vi "FTW-Test.vi"() -> ()   [LabVIEW 2015]
uses:
  src/time/FTW-Time-DisplayFormat-Timestamp.ctl
  src/json/core/FTW-JSON-Core-Type.ctl
  src/reflection/FTW-Reflection-Types.ctl
  src/error/FTW-ERR-ExceptionType.ctl
  src/time/FTW-Time-RelativeTimer.vi
  codegen/xnode/json/fetch/FTW-JSON-Core-GetFlattenedValue.vi
  src/error/FTW-ERR-ThrowInvalidReferenceError.vi
  src/json/core/FTW-JSON-Core-ElementType.vi
  codegen/xnode/FTW-Dataflow-Synchronizer.xnode
  codegen/xnode/FTW-JSON-Fetch.xnode
  codegen/xnode/FTW-Array-Shuffle.xnode
  src/json/FTW-JSON-Type.ctl
panel:
  out "Results":string
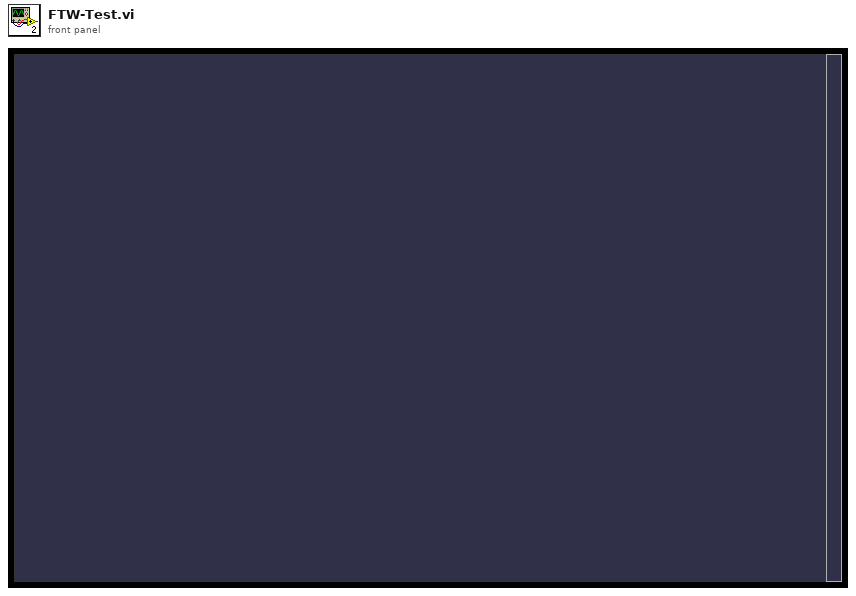
[diagram p1: front panel]
types:
  T1 = typedef "FTW-Time-DisplayFormat-Timestamp.ctl" = enum16{"YYYY-MM-DDT00:00:00.000Z (ISO-8601)", "YYYY-MM-DDT00-00-00Z (Simple ISO-8601)", "YYYY-MM-DD"}
  T2 = cluster{"Randomize Test Order":bool, "Tests Directory":path, "Test Configuration":cluster{"Default":cluster{"Enable":bool, "Iterations":i32}}, "Test Configuration":string, "Test Worker Pool Size":i32}
  T3 = typedef "FTW-Type-JSON.ctl" = refnum<data-value>
  T4 = enum32{"invalid app kind", "Development System", "Run Time System", "Student Edition", "Embedded LabVIEW", "Evaluation", "Custom"}
  T5 = enum32{"invalid CPU target", "Motorola 68K", "PowerPC", "Intel x86", "SPARC", "PA-RISC", "MIPS", "Alpha", "ARM", "AMD/Intel x64"}
  T6 = typedef "FTW-JSON-Core-Type.ctl" = enum8{"Object", "Array", "String", "Integer", "Floating Point", "true", "false", "null", "undefined"}
  T7 = typedef "FTW-ERR-ExceptionType.ctl" = enum16{"OK", "Info", "Warning", "Error"}
  T8 = cluster{"Execute?":bool, "TestName":string, "MinTime":dbl, "MeanTime":dbl, "MaxTime":dbl, "Runs":i32, "Result":T7, "Hint":string, "TotalTime":dbl, "Passes":i32, "Warnings":i32, "Failures":i32}
  T9 = enum32{"Bad", "Idle", "Run top level", "Running"}
  T10 = cluster{"VIRef":refnum<vi>, "TestName":string, "TestInstance":i32, "TestPoolSize":i32, "TestID":i32}
  T11 = cluster{"Color":u32, "Text":string, "Comment":string}[]
  T12 = typedef "FTW-Type-Regex.ctl" = refnum<data-value>
  T13 = cluster{"Color":u32, "Text":string, "Comment":string}
  T14 = cluster{u32, "offset past match":u32, "Color":u32}[]
  T15 = cluster{"VIRef":refnum<vi>, "TestName":string, "TestInstance":i32, "TestPoolSize":i32, "TestID":i32}[]
  T16 = cluster{"Result":T7, "TestID":i32, "ElapsedTime":dbl}
  T17 = cluster{"Execute?":bool, "TestName":string, "MinTime":dbl, "MeanTime":dbl, "MaxTime":dbl, "Runs":i32, "Result":T7, "Hint":string, "TotalTime":dbl, "Passes":i32, "Warnings":i32, "Failures":i32}[]
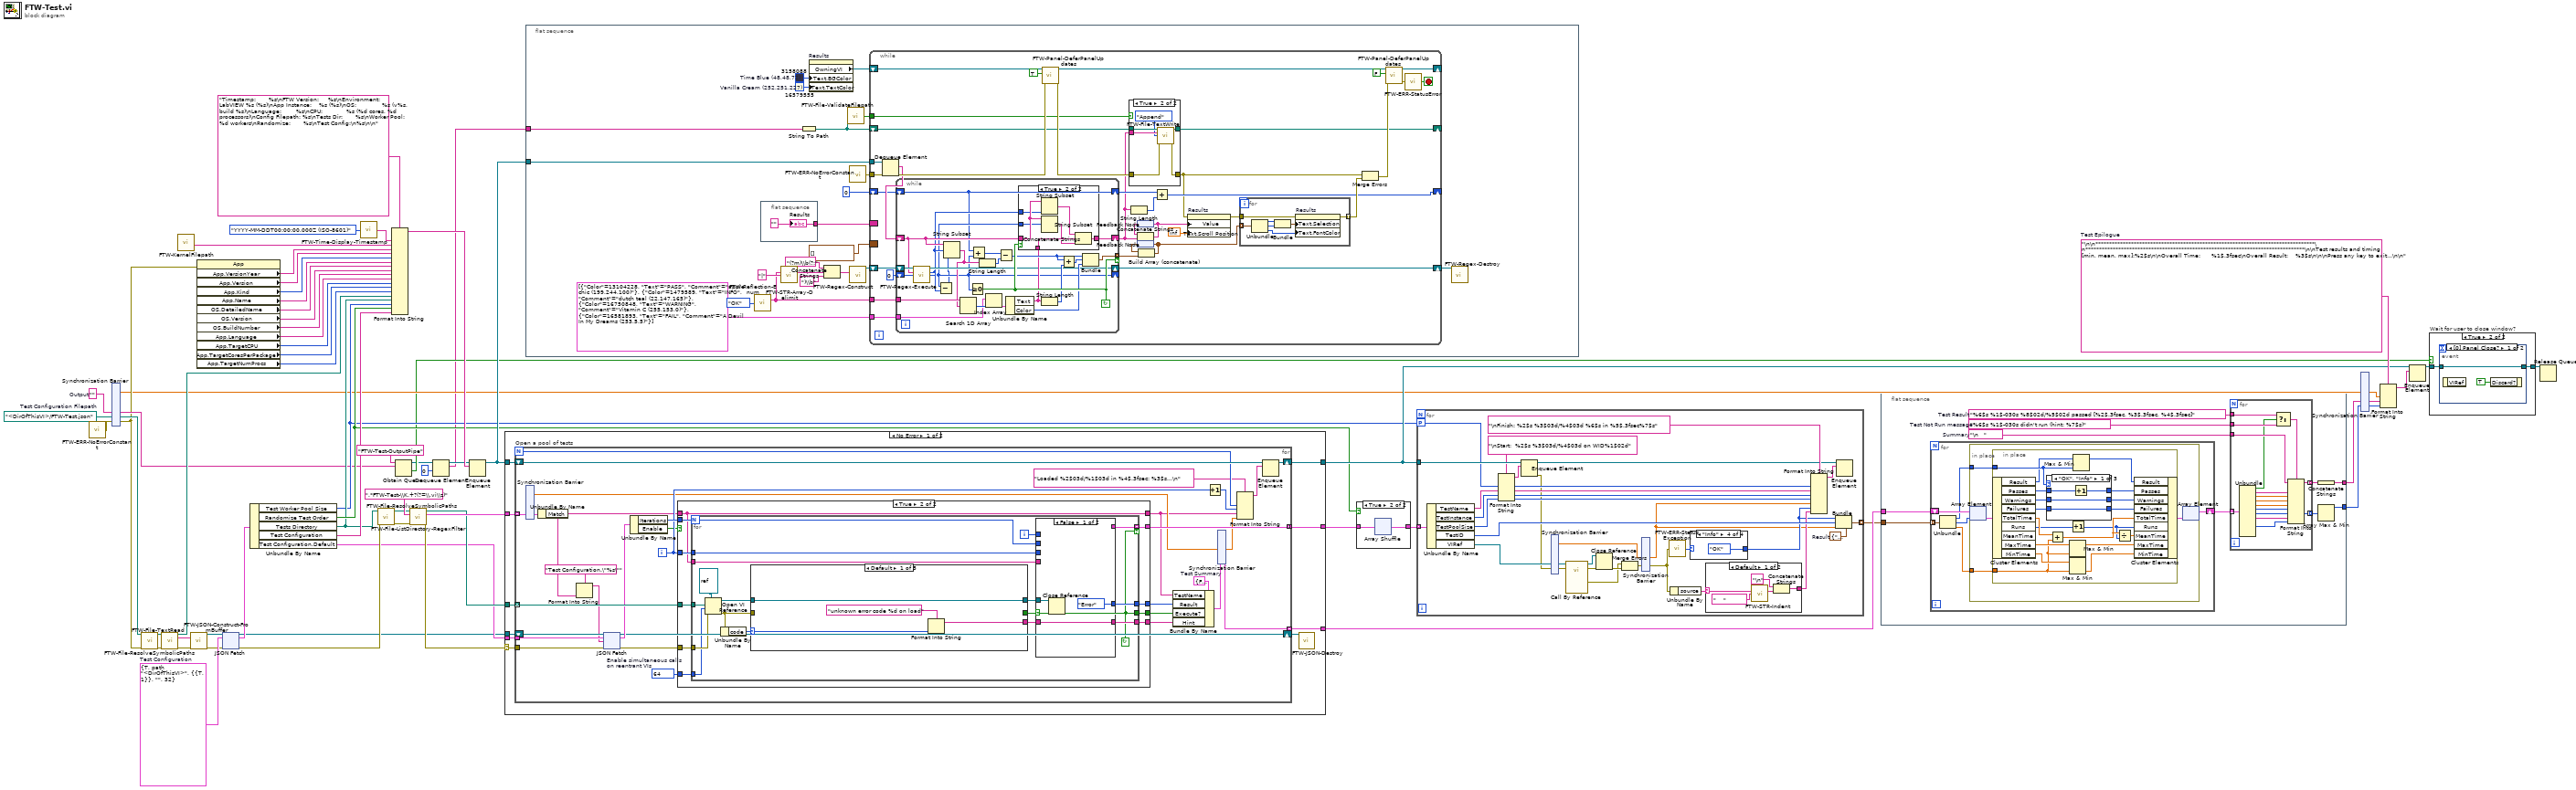
[diagram p0: block diagram]
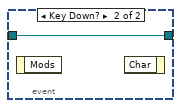
[diagram p3: hidden frame]
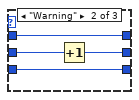
[diagram p4: hidden frame]
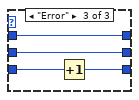
[diagram p5: hidden frame]
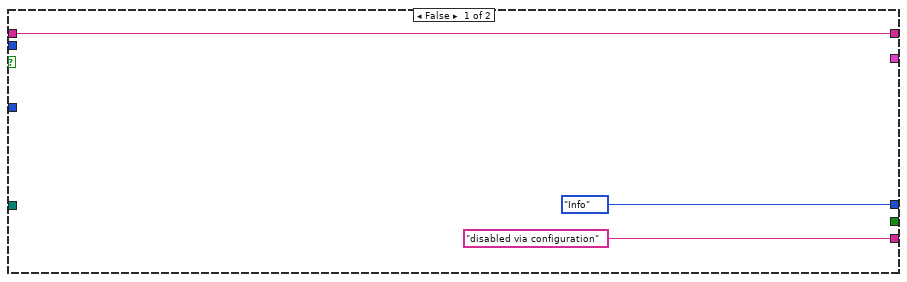
[diagram p7: hidden frame]
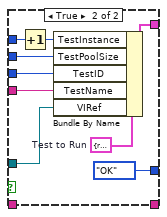
[diagram p8: hidden frame]
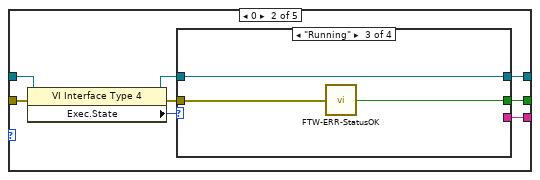
[diagram p9: hidden frame]
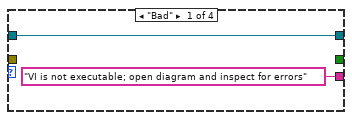
[diagram p10: hidden frame]
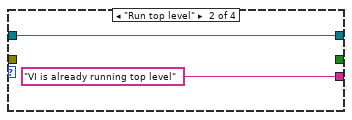
[diagram p11: hidden frame]
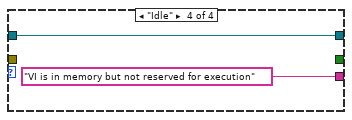
[diagram p12: hidden frame]
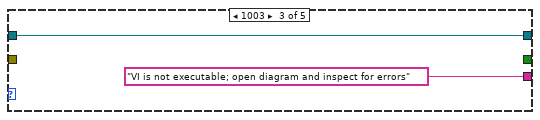
[diagram p13: hidden frame]
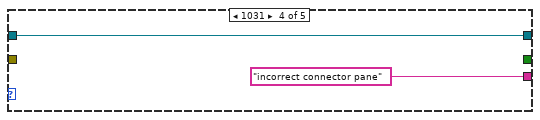
[diagram p14: hidden frame]
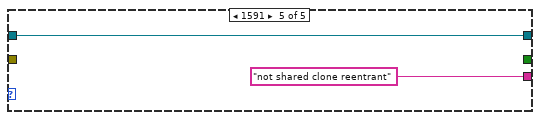
[diagram p15: hidden frame]
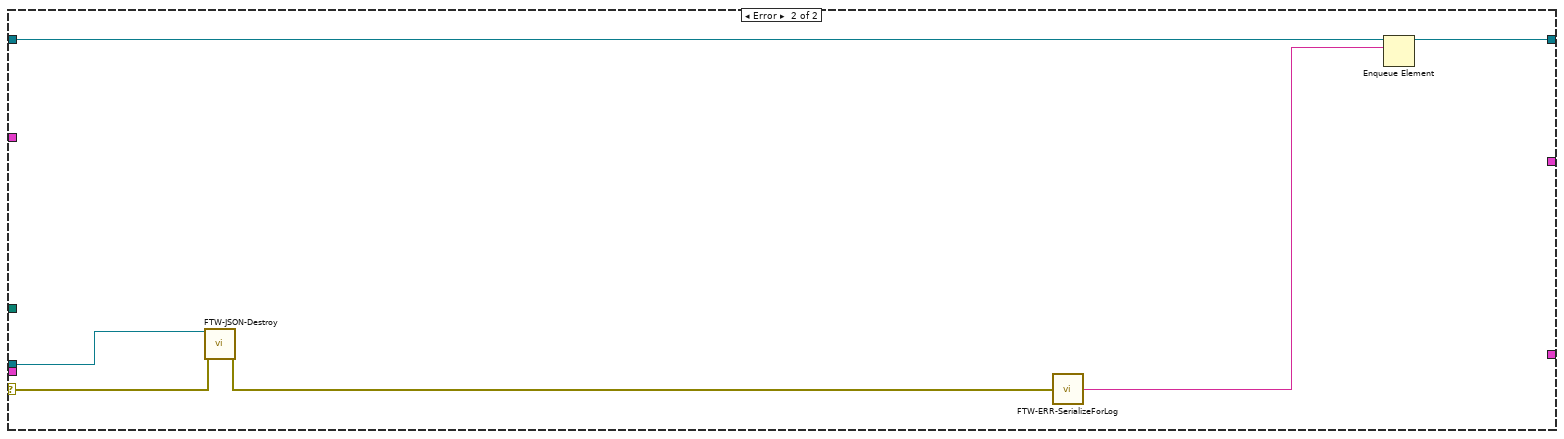
[diagram p16: hidden frame]
diagram:
  w57 = "\n\n********************************************************************************\n********************************************************************************\n\nTest results and timing [min, mean, max]:%2$s\n\nOverall Time:      %1$.3fsec\nOverall Result:    %3$s\n\n\nPress any key to exit...\n\n"  # Test Epilogue
  w25 = path "<DirOfThisVI>/FTW-Test.json"  # Test Configuration Filepath
  w8 = T2 {"Randomize Test Order"=TRUE, "Tests Directory"=path "<DirOfThisVI>", "Test Configuration"={"Default"={"Enable"=TRUE, "Iterations"=1}}, "Test Configuration"="", "Test Worker Pool Size"=32}  # Test Configuration
  w27 = ""  # Output
  n1 = call "FTW-ERR-NoErrorConstant.vi"() -> ("no error"=w23:errorcluster)
  n2 = xnode "Synchronization Barrier"("Synchronized Signal 1"=w27, "Synchronized Signal 2"=w25, "Synchronized Signal 3"=w23) -> ("High-Resolution Timer"=w20:dbl, "Output out"=w26:string, "Test Configuration Filepath out"=w24:path, "no error out"=w22:errorcluster)  [unwired: 1 in, 1 out]
  n3 = call "FTW-File-ResolveSymbolicPaths.vi"("Unresolved Path"=w24, "error in"=w22) -> ("Resolved Path"=w42:path, "error out"=w58:errorcluster)  [unwired: 12 in]
  n4 = call "FTW-File-TextRead.vi"("Filepath"=w42, "error in"=w58) -> ("Filepath out"=w35:path, "Text"=w3:string, "error out"=w5:errorcluster)  [unwired: 11 in]
  n5 = call "FTW-KernelFilepath.vi"() -> ("Expected FTW Kernel ABI Version"=w33:string)  [unwired: 9 in, 2 out]
  n6 = call "FTW-JSON-Construct-FromBuffer.vi"("JSON String (UTF-8)"=w3, "error in"=w5) -> ("JSON"=w2:T3, "error out"=w4:errorcluster)  [unwired: 12 in]
  n7 = property class="App"(error in=w22) -> ("App.VersionYear"=w54:string, "App.Version"=w52:string, "App.Kind"=w44:T4, "App.Name"=w43:string, "OS.DetailedName"=w53:string, "OS.Version"=w51:string, "OS.BuildNumber"=w50:string, "App.Language"=w49:string, "App.TargetCPU"=w48:T5, "App.TargetCoresPerPackage"=w47:i32, "App.TargetNumProcs"=w45:i32)  [unwired: 1 in, 2 out]
  n8 = xnode "JSON Fetch"("JSON"=w2, "Element Type and Default Value"=w8, "error in"=w4) -> ("JSON out"=w1:T3, "Value"=w7:T2, "error out"=w21:errorcluster)  [unwired: 2 in, 2 out]
  n9 = Unbundle By Name(w7) -> ("Test Worker Pool Size"=w30:i32, "Randomize Test Order"=w34:bool, "Tests Directory"=w31:path, "Test Configuration"=w36:string, "Test Configuration.Default"=w6:cluster{"Enable":bool, "Iterations":i32})
  n10 = call "FTW-Time-Display-Timestamp.vi"("Format"=FTW-Time-DisplayFormat-Timestamp."YYYY-MM-DDT00:00:00.000Z (ISO-8601)") -> ("Formatted Timestamp"=w40:string)  [unwired: 3 in]
  n11 = call "FTW-File-ResolveSymbolicPaths.vi"("Unresolved Path"=w31, "error in"=w21) -> ("Resolved Path"=w32:path, "error out"=w62:errorcluster)  [unwired: 12 in]
  n12 = Format Into String(format string="Timestamp:       %s\nFTW Version:     %s\nEnvironment:     LabVIEW %s (%s)\nApp Instance:    %s (%s)\nOS:              %s (v%s, build %s)\nLanguage:        %s\nCPU:             %s (%d cores, %d processors)\nConfig Filepath: %s\nTests Dir:       %s\nWorker Pool:     %d workers\nRandomize:       %s\nTest Config:\n%s\n\n", w40, w33, w54, w52, w44, w43, w53, w51, w50, w49, w48, w47, w45, w35, w31, w30, w34, w36) -> (resulting string=w41:string)  [unwired: 2 in, 1 out]
  n13 = Obtain Queue(name (unnamed)="FTW-Test-OutputPipe", element data type=w26) -> (queue out=w11:refnum<queue>, created new?=w13:bool)  [unwired: 3 in, 1 out]
  n14 = call "FTW-File-ListDirectory-RegexFilter.vi"("Directory to Search"=w32, "Filename Regex Filter"=".*FTW-Test-\\K.+?(?=\\.vi\\z)", "error in"=w62) -> ("Matching Filepaths"=w64:path[], "Regex Results"=w65:cluster{"Match":string, "Submatches":string[]}[], "error out"=w56:errorcluster)  [unwired: 9 in, 1 out]
  n15 = Dequeue Element(queue=w11, timeout in ms (-1)=0) -> (queue out=w10:refnum<queue>, element=w9:string)  [unwired: 1 in, 2 out]
  n16 = Enqueue Element(queue=w10, element=w41) -> (queue out=w55:refnum<queue>)  [unwired: 2 in, 2 out]
  n17 = case shown="No Error" w56 {
    selector: w56 -> [w72 w237]
    tunnel: w65 -> [w76 _]
    tunnel: w64 -> [w75 _]
    tunnel: [w68 _] -> w37
    tunnel: w1 -> [w73 w238]
    tunnel: [w71 _] -> w61
    tunnel: w55 -> [w70 w239]
    tunnel: [w69 w241] -> w38
    tunnel: w6 -> [w74 _]
    frame No Error {
      n18 = for "Open a pool of tests" {
        N -> [w102]
        tunnel: w72 -> [w87]
        tunnel: [w100] -> w68 mode=concatenating
        tunnel: w76 -> [w93] mode=indexing
        tunnel: w75 -> [w108] mode=indexing
        tunnel: [w89] -> w71 mode=indexing
        shift-right: [w99] -> w69
        shift-left: w70 -> [w104]
        shift-right: [w82] -> w67
        shift-left: w73 -> [w85]
        tunnel: w74 -> [w84]
        i -> [w101]
        w98 = 64  # Enable simultaneous calls on reentrant VIs
        w105 = T8 {"Execute?"=FALSE, "TestName"="", "MinTime"=inf, "MeanTime"=0.0, "MaxTime"=-inf, "Runs"=0, "Result"=enum."OK", "Hint"="", "TotalTime"=0.0, "Passes"=0, "Warnings"=0, "Failures"=0}  # Test Summary
        n19 = xnode "Synchronization Barrier"("Synchronized Signal 1"=w93) -> ("High-Resolution Timer"=w91:dbl, "Regex Result out"=w92:cluster{"Match":string, "Submatches":string[]})  [unwired: 1 in, 1 out]
        n20 = Unbundle By Name(w92) -> ("Match"=w77:string)
        n21 = Format Into String(format string="Test Configuration.\"%s\"", w77) -> (resulting string=w80:string)  [unwired: 2 in, 1 out]
        n22 = xnode "JSON Fetch"("JSON"=w85, "Element Type and Default Value"=w84, "Element Path"=w80, "error in"=w87) -> ("JSON out"=w82:T3, "Value"=w83:cluster{"Enable":bool, "Iterations":i32}, "error out"=w86:errorcluster)  [unwired: 1 in, 2 out]
        n23 = Unbundle By Name(w83) -> ("Iterations"=w106:i32, "Enable"=w96:bool)
        n24 = case shown="True" w96 {
          tunnel: w108 -> [_ w179]
          tunnel: w98 -> [_ w178]
          tunnel: [_ w177] -> w100
          tunnel: w101 -> [_ w176]
          tunnel: ["disabled via configuration" w175] -> w107
          tunnel: w106 -> [_ w174]
          tunnel: w86 -> [_ w173]
          tunnel: [FTW-ERR-ExceptionType."Info" ("Result") w172] -> w78
          tunnel: [_ w171] -> w95
          tunnel: [w167 w170] -> w79
          tunnel: w77 -> [w167 w170]
          frame False {
          }
          frame True {
            n25 = for {
              N: w174 -> [w188]
              tunnel: w173 -> [w196]
              tunnel: w179 -> [w195]
              tunnel: w178 -> [w194]
              tunnel: w170 -> [w190]
              tunnel: [w187] -> w177 mode=indexing if=w180
              tunnel: [w183] -> w175
              tunnel: w176 -> [w182]
              tunnel: [w181] -> w172
              tunnel: [w180] -> w171
              i -> [w189]
              stop <- w180 continue-if-true
              n26 = Open VI Reference(type specifier VI Refnum (for type only)=refnum<vi> refnum, vi path=w195, options=w194, error in (no error)=w196) -> (vi reference=w186:refnum<vi>, error out=w192:errorcluster)  [unwired: 2 in]
              n27 = Unbundle By Name(w192) -> ("code"=w191:i32)
              n28 = case shown="Default" w191 {
                selector: w191 -> [w211 _ _ _ _]
                tunnel: w186 -> [w209 w220 w230 w232 w234]
                tunnel: w192 -> [_ w219 _ _ _]
                tunnel: [_ w216 _ _ _] -> w180
                tunnel: [w210 w214 "VI is not executable; open diagram and inspect for errors" "incorrect connector pane" "not shared clone reentrant"] -> w184
                tunnel: [w209 w213 w230 w232 w234] -> w185
                frame Default {
                  n29 = Format Into String(format string="unknown error code %d on load", w211) -> (resulting string=w210:string)  [unwired: 2 in, 1 out]
                }
                frame 0 {
                  n30 = property class="VI Interface Type 4"(reference=w220, error in=w219) -> (reference out=w217:refnum<vi>, error out=w218:errorcluster, "Exec.State"=w215:T9)
                  n31 = case shown="\"Running\"" w215 {
                    tunnel: w218 -> [_ _ w226 _]
                    tunnel: w217 -> [w221 w223 w227 w229]
                    tunnel: [_ _ w225 _] -> w216
                    tunnel: ["VI is not executable; open diagram and inspect for errors" "VI is already running top level" _ "VI is in memory but not reserved for execution"] -> w214
                    tunnel: [w221 w223 w227 w229] -> w213
                    frame "Bad" {
                    }
                    frame "Run top level" {
                    }
                    frame "Running" {
                      n32 = call "FTW-ERR-StatusOK.vi"("error to check"=w226) -> ("Status OK?"=w225:bool)
                    }
                    frame "Idle" {
                    }
                  }
                }
                frame 1003 {
                }
                frame 1031 {
                }
                frame 1591 {
                }
              }
              n33 = case shown="False" w180 {
                tunnel: w185 -> [w199 w208]
                tunnel: w190 -> [_ w202]
                tunnel: w189 -> [_ w207]
                tunnel: w188 -> [_ w205]
                tunnel: [_ w206] -> w187
                tunnel: w184 -> [w198 _]
                tunnel: [w198 _] -> w183
                tunnel: w182 -> [_ w204]
                tunnel: [FTW-ERR-ExceptionType."Error" ("Result") FTW-ERR-ExceptionType."OK" ("Result")] -> w181
                frame False {
                  n34 = Close Reference(reference=w199) -> ()  [unwired: 1 in, 1 out]
                }
                frame True {
                  w203 = T10 {"VIRef"=refnum, "TestName"="", "TestInstance"=0, "TestPoolSize"=0, "TestID"=0}  # Test to Run
                  n35 = Increment(x=w207) -> (x+1=w201:i32)
                  n36 = Bundle By Name(cluster=w203, "TestInstance"=w201, "TestPoolSize"=w205, "TestID"=w204, "TestName"=w202, "VIRef"=w208) -> (w206:T10)
                }
              }
            }
          }
        }
        n37 = Bundle By Name(cluster=w105, "TestName"=w79, "Result"=w78, "Execute?"=w95, "Hint"=w107) -> (w90:T8)
        n38 = Increment(x=w101) -> (x+1=w97:i32)
        n39 = xnode "Synchronization Barrier"("Upstream Timer Value"=w91, "Synchronized Signal 3"=w90) -> ("Elapsed Time"=w88:dbl, "Test Summary out"=w89:T8)  [unwired: 1 out]
        n40 = Format Into String(format string="Loaded %2$03d/%1$03d in %4$.3fsec: %3$s...\n", w102, w97, w79, w88) -> (resulting string=w103:string)  [unwired: 2 in, 1 out]
        n41 = Enqueue Element(queue=w104, element=w103) -> (queue out=w99:refnum<queue>)  [unwired: 2 in, 2 out]
      }
      n42 = call "FTW-JSON-Destroy.vi"("JSON"=w67) -> ()  [unwired: 14 in, 1 out]
    }
    frame Error {
      n43 = call "FTW-JSON-Destroy.vi"("JSON"=w238, "error in"=w237) -> ("error out"=w236:errorcluster)  [unwired: 13 in]
      n44 = call "FTW-ERR-SerializeForLog.vi"("error in"=w236) -> ("Serialized Error"=w240:string)
      n45 = Enqueue Element(queue=w239, element=w240) -> (queue out=w241:refnum<queue>)  [unwired: 2 in, 2 out]
    }
  }
  n46 = flat-sequence {
    tunnel: w55 -> [w262]
    tunnel: w9 -> [w244]
    frame #0 {
      w258 = u32 16579555  # Vanilla Cream (252,251,227)
      w259 = u32 3158088  # Time Blue (48,48,72)
      n47 = call "FTW-Reflection-Enum.vi"("Enum"=FTW-ERR-ExceptionType."OK" ("Exception")) -> ("Enum Items"=w253:string[])  [unwired: 12 in, 2 out]
      n48 = flat-sequence {
        tunnel: [w263] -> w251
        frame #0 {
          w263 = "" ("Results")
          "Results" <- w263
        }
      }
      n49 = call "FTW-STR-Array-Delimit.vi"("Array of Strings"=w253, "Delimiter"="|") -> ("Delimited String"=w254:string)  [unwired: 13 in]
      n50 = String To Path(string=w244) -> (path=w242:path)
      n51 = property on="Results" class="Str"("Text.BGColor"=w259, "Text.TextColor"=w258) -> ("OwningVI"=w257:refnum<vi>)  [unwired: 2 in, 2 out]
      n52 = Concatenate Strings("(?m)\\b(?:" ("string"), w254, ")\\b" ("string")) -> (w247:string)
      n53 = call "FTW-File-ValidateFilepath.vi"("Filepath"=w242) -> ("Valid?"=w243:bool)
      n54 = call "FTW-ERR-NoErrorConstant.vi"() -> ("no error"=w248:errorcluster)
      n55 = call "FTW-Regex-Construct.vi"("Regular Expression"=w247) -> ("Regex"=w246:T12)  [unwired: 13 in, 1 out]
      n56 = while {
        border: cluster{u32, "offset past match":u32, u32}[] [] -> [_]
        border: w251 -> [_]
        tunnel: w253 -> [w296]
        tunnel: T11 [{"Color"=13104228, "Text"="PASS", "Comment"="apple chic (199,244,100)"}, {"Color"=1479589, "Text"="INFO", "Comment"="dutch teal (22,147,165)"}, {"Color"=16750848, "Text"="WARNING", "Comment"="Vitamin C (255,153,0)"}, {"Color"=16581893, "Text"="FAIL", "Comment"="A Devil In My Dreams (253,5,5)"}] -> [w286]
        shift-right: [w285] -> _
        shift-left: w257 -> [w295]
        tunnel: w262 -> [w298]
        tunnel: w248 -> [w281]
        shift-right: [w276] -> _
        shift-left: 0 ("length") -> [w269]
        shift-right: [w273] -> w245
        shift-left: w246 -> [w274]
        tunnel: w243 -> [w267]
        shift-right: [w265] -> _
        shift-left: w242 -> [w266]
        stop <- w284 stop-if-true
        n57 = Dequeue Element(queue=w298, error in (no error)=w281) -> (element=w283:string, error out=w297:errorcluster)  [unwired: 1 in, 2 out]
        n58 = while {
          shift-right: [w316] -> _
          shift-left: 0 ("offset past match") -> [w321]
          tunnel: [w334] -> w292 mode=indexing if=w332
          tunnel: w296 -> [w336]
          shift-right: [w333] -> w264
          shift-left: w283 -> [w319]
          tunnel: w286 -> [w330]
          shift-right: [w320] -> w273
          shift-left: w274 -> [w322]
          shift-right: [w314] -> w268
          shift-left: w269 -> [w314]
          stop <- w332 continue-if-true
          n59 = call "FTW-Regex-Execute.vi"("Regex"=w322, "Subject String"=w319, "Starting Offset"=w321) -> ("Regex out"=w320:T12, "Whole Match Begin"=w317:i32, "Offset after Match"=w316:i32)  [unwired: 7 in, 3 out]
          n60 = Subtract(x=w316, y=w317) -> (x-y=w315:i32)
          n61 = String Subset(string=w319, offset (0)=w317, length (rest)=w315) -> (substring=w318:string)
          n62 = Search 1D Array(1D array=w336, element=w318) -> (index of element=w331:i32)  [unwired: 1 in]
          n63 = Greater Or Equal To 0?(x=w316) -> (x >= 0?=w332:bool)
          n64 = Add(x=w314, y=w316) -> (x+y=w335:i32)
          n65 = String Length(string=w318) -> (length=w329:i32)
          n66 = Index Array(array=w330, index=w331) -> (element=w325:T13)
          n67 = Subtract(x=w335, y=w329) -> (x-y=w328:i32)
          n68 = Unbundle By Name(w325) -> ("Text"=w324:string, "Color"=w323:u32)
          n69 = case shown="True" w332 {
            tunnel: [w337 w344] -> w333
            tunnel: w324 -> [_ w342]
            tunnel: w319 -> [w337 w341]
            tunnel: w317 -> [_ w338]
            tunnel: w316 -> [_ w340]
            frame False {
            }
            frame True {
              n70 = String Subset(string=w341, length (rest)=w338) -> (substring=w343:string)  [unwired: 1 in]
              n71 = String Subset(string=w341, offset (0)=w340) -> (substring=w339:string)  [unwired: 1 in]
              n72 = Concatenate Strings(w343, w342, w339) -> (w344:string)
            }
          }
          n73 = String Length(string=w324) -> (length=w326:i32)
          n74 = Add(x=w328, y=w326) -> (x+y=w327:i32)
          n75 = Bundle(w328, w327, "Color"=w323) -> (w334:cluster{i32, i32, "Color":u32})  [unwired: 1 in]
        }
        n76 = call "FTW-Panel-DeferPanelUpdates.vi"("error in"=w297, "Defer?"=TRUE, "VI Ref"=w295) -> ("error out"=w271:errorcluster, "VI Ref out"=w288:refnum<vi>)  [unwired: 7 in]
        n77 = case shown="True" w267 {
          tunnel: w271 -> [w299 w306]
          tunnel: [w299 w305] -> w270
          tunnel: w266 -> [w300 w304]
          tunnel: [w300 w303] -> w265
          tunnel: w264 -> [_ w302]
          frame False {
          }
          frame True {
            n78 = call "FTW-File-TextWrite.vi"("Filepath"=w304, "Text to Write"=w302, "Mode"=enum16{"Overwrite", "Append"}."Append", "error in"=w306) -> ("Filepath out"=w303:path, "error out"=w305:errorcluster)  [unwired: 10 in]
          }
        }
        n79 = String Length(string=w264) -> (length=w280:i32)
        n80 = feedback #1() -> (w290:string)
        n81 = Concatenate Strings(w290, w264) -> (w291:string)
        n82 = feedback-in #1(w291) -> ()
        n83 = feedback #2() -> (w293:cluster{u32, "offset past match":u32, u32}[])
        n84 = Build Array (concatenate)(w293, w292) -> (w272:T14)
        n85 = feedback-in #2(w272) -> ()
        n86 = Add(x=w268, y=w280) -> (x+y=w276:i32)
        n87 = property on="Results" class="Str"(error in=w270, "Value"=w291, "Text.Scroll Position"=inf) -> (error out=w279:errorcluster)  [unwired: 1 in, 1 out]
        n88 = for {
          tunnel: w272 -> [w313] mode=indexing
          tunnel: w279 -> [w308]
          tunnel: [w307] -> w278 mode=indexing
          n89 = Unbundle(w313) -> (w311:u32, "offset past match"=w310:u32, "Color"=w312:u32)
          n90 = Bundle(w311, "offset past match"=w310) -> (w309:cluster{u32, "offset past match":u32})  [unwired: 1 in]
          n91 = property on="Results" class="Str"(error in=w308, "Text.Selection"=w309, "Text.FontColor"=w312) -> (error out=w307:errorcluster)  [unwired: 1 in, 1 out]
        }
        n92 = Merge Errors(w270, w278) -> (w277:errorcluster)
        n93 = call "FTW-Panel-DeferPanelUpdates.vi"("error in"=w277, "Defer?"=FALSE, "VI Ref"=w288) -> ("error out"=w282:errorcluster, "VI Ref out"=w285:refnum<vi>)  [unwired: 7 in]
        n94 = call "FTW-ERR-StatusError.vi"("error to check"=w282) -> ("Error?"=w284:bool)
      }
      n95 = call "FTW-Regex-Destroy.vi"("Regex"=w245) -> ()  [unwired: 14 in, 1 out]
    }
  }
  n96 = case shown="True" w34 {
    tunnel: [w345 w346] -> w28
    tunnel: w37 -> [w345 w347]
    frame False {
    }
    frame True {
      n97 = xnode "Array Shuffle"("Array"=w347) -> ("Shuffled Array"=w346:T15)
    }
  }
  n98 = for {
    tunnel: w28 -> [w393] mode=indexing
    workers-P: w30 -> [w373]
    tunnel: [w389] -> w29 mode=indexing
    tunnel: w38 -> [w392]
    w378 = T16 {"Result"=enum."OK", "TestID"=0, "ElapsedTime"=0.0}  # Result
    n99 = Unbundle By Name(w393) -> ("TestName"=w376:string, "TestInstance"=w375:i32, "TestPoolSize"=w374:i32, "TestID"=w390:i32, "VIRef"=w372:refnum<vi>)
    n100 = Format Into String(format string="\nStart:  %2$s %3$03d/%4$03d on WID%1$02d", w373, w376, w375, w374) -> (resulting string=w391:string)  [unwired: 2 in, 1 out]
    n101 = Enqueue Element(queue=w392, element=w391) -> (queue out=w379:refnum<queue>, error out=w371:errorcluster)  [unwired: 2 in, 1 out]
    n102 = xnode "Synchronization Barrier"("Synchronized Signal 1"=w372, "Synchronized Signal 2"=w371) -> ("High-Resolution Timer"=w367:dbl, "VIRef out"=w370:refnum<vi>, "error out out"=w369:errorcluster)  [unwired: 1 in, 1 out]
    n103 = call-by-ref "?"(reference=w370, error in=w369) -> (reference out=w388:refnum<vi>, error out=w387:errorcluster, "Test Result"=w385:errorcluster)
    n104 = Close Reference(reference=w388, error in (no error)=w387) -> (error out=w386:errorcluster)
    n105 = Merge Errors(w385, w386) -> (w366:errorcluster)
    n106 = xnode "Synchronization Barrier"("Upstream Timer Value"=w367, "Synchronized Signal 1"=w366) -> ("Elapsed Time"=w368:dbl, "error IO out"=w365:errorcluster)  [unwired: 1 out]
    n107 = call "FTW-ERR-StatusException.vi"("error to check"=w365) -> ("Exception"=w380:T7)
    n108 = Unbundle By Name(w365) -> ("source"=w384:string)
    n109 = case shown="\"Info\"" w380 {
      selector: w380 -> [w404 w405 w406 _]
      tunnel: [w404 w405 w406 FTW-ERR-ExceptionType."OK" ("Result")] -> w377
      frame "OK" {
      }
      frame "Warning" {
      }
      frame "Error" {
      }
      frame "Info" {
      }
    }
    n110 = case shown="Default" w384 {
      selector: w384 -> [w410 w413]
      tunnel: [w411 w413] -> w383
      frame Default {
        n111 = call "FTW-STR-Indent.vi"("String"=w410, "Indentation Characters"="    ") -> ("Indented String"=w409:string)  [unwired: 13 in]
        n112 = Concatenate Strings("\n", w409) -> (w411:string)
      }
      frame "" {
      }
    }
    n113 = Format Into String(format string="\nFinish: %2$s %3$03d/%4$03d %6$s in %5$.3fsec%7$s", w373, w376, w375, w374, w368, w377, w383) -> (resulting string=w394:string)  [unwired: 2 in, 1 out]
    n114 = Bundle(cluster=w378, "Result"=w377, "TestID"=w390, "ElapsedTime"=w368) -> (w389:T16)
    n115 = Enqueue Element(queue=w379, element=w394) -> ()  [unwired: 2 in, 3 out]
  }
  n116 = flat-sequence {
    tunnel: w29 -> [w423]
    tunnel: w61 -> [w422]
    tunnel: [w416] -> w16
    tunnel: [w415] -> w18
    frame #0 {
      w414 = "\n   "  # Summary
      w417 = "%6$s %1$-030s %8$02d/%5$02d passed [%2$.3fsec, %3$.3fsec, %4$.3fsec]"  # Test Result
      w418 = "%6$s %1$-030s didn't run (hint: %7$s)"  # Test Not Run message
      n117 = for {
        tunnel: w423 -> [w442] mode=indexing
        shift-right: [w443] -> w421
        shift-left: w422 -> [w444]
        n118 = Unbundle(w442) -> ("Result"=w441:T7, "TestID"=w440:i32, "ElapsedTime"=w439:dbl)
        n119 = in-place {
          in-place-border: w439 -> [w446]
          in-place-border: w441 -> [w445]
          n120 = in-place-array #3(w444, w440) -> (w448:T8)
          n121 = in-place {
            in-place-border: w446 -> [w459]
            in-place-border: w445 -> [w457]
            n122 = in-place-cluster #4(w448) -> ("Result"=w449:T7, "Passes"=w456:i32, "Warnings"=w453:i32, "Failures"=w452:i32, "TotalTime"=w467:dbl, "Runs"=w466:i32, "MaxTime"=w462:dbl, "MinTime"=w460:dbl)  [unwired: 1 out]
            n123 = case shown="\"OK\", \"Info\"" w457 {
              tunnel: w456 -> [w471 w475 w479]
              tunnel: [w468 w475 w479] -> w455
              tunnel: [w470 w472 w478] -> w454
              tunnel: w453 -> [w470 w474 w478]
              tunnel: [w469 w473 w476] -> w451
              tunnel: w452 -> [w469 w473 w477]
              frame "OK", "Info" {
                n124 = Increment(x=w471) -> (x+1=w468:i32)
              }
              frame "Warning" {
                n125 = Increment(x=w474) -> (x+1=w472:i32)
              }
              frame "Error" {
                n126 = Increment(x=w477) -> (x+1=w476:i32)
              }
            }
            n127 = Add(x=w467, y=w459) -> (x+y=w465:dbl)
            n128 = Max & Min(x=w462, y=w459) -> (max(x,y)=w461:dbl)  [unwired: 1 out]
            n129 = Max & Min(x=w460, y=w459) -> (min(x,y)=w458:dbl)  [unwired: 1 out]
            n130 = Increment(x=w466) -> (x+1=w464:i32)
            n131 = Max & Min(x=w449, y=w457) -> (max(x,y)=w450:u16)  [unwired: 1 out]
            n132 = Divide(x=w465, y=w464) -> (x/y=w463:dbl)
            n133 = in-place-cluster #4("Result"=w450, "Passes"=w455, "Warnings"=w454, "Failures"=w451, "TotalTime"=w465, "Runs"=w464, "MeanTime"=w463, "MaxTime"=w461, "MinTime"=w458) -> (w447:T8)
          }
          n134 = in-place-array #3(w447) -> (w443:T17)  [unwired: 1 out]
        }
      }
      n135 = for {
        tunnel: w421 -> [w428] mode=indexing
        tunnel: [w438] -> w420 mode=indexing
        tunnel: w417 -> [w433]
        tunnel: w418 -> [w432]
        tunnel: [w425] -> w419 mode=indexing
        tunnel: w414 -> [w429]
        n136 = Unbundle(w428) -> ("Execute?"=w426:bool, "TestName"=w437:string, "MinTime"=w436:dbl, "MeanTime"=w435:dbl, "MaxTime"=w434:dbl, "Runs"=w430:i32, "Result"=w425:T7, "Hint"=w427:string, "Passes"=w424:i32)  [unwired: 3 out]
        n137 = Select(t=w433, s=w426, f=w432) -> (s? t:f=w431:string)
        n138 = Format Into String(format string=w431, initial string=w429, w437, w436, w435, w434, w430, w425, w427, w424) -> (resulting string=w438:string)  [unwired: 1 in, 1 out]
      }
      n139 = Concatenate Strings(w420) -> (w415:string)
      n140 = Array Max & Min(array=w419) -> (max value=w416:T7)  [unwired: 3 out]
    }
  }
  n141 = xnode "Synchronization Barrier"("Upstream Timer Value"=w20, "Synchronized Signal 1"=w18, "Synchronized Signal 2"=w16) -> ("Elapsed Time"=w19:dbl, "out"=w17:string, "out"=w15:T7)  [unwired: 1 out]
  n142 = Format Into String(format string=w57, w19, w17, w15) -> (resulting string=w63:string)  [unwired: 2 in, 1 out]
  n143 = Enqueue Element(queue=w38, element=w63) -> (queue out=w60:refnum<queue>)  [unwired: 2 in, 2 out]
  n144 = case "Wait for user to close window?" shown="True" w13 {
    tunnel: w60 -> [w480 w482]
    tunnel: [w480 w481] -> w59
    frame False {
    }
    frame True {
      n145 = event shown="[0] Panel Close?" {
        selector: _ -> [_ _]
        dyn-events: _ -> [_ _]
        timeout: _ -> [_ _]
        tunnel: w482 -> [w483 w485]
        tunnel: [w483 w485] -> w481
        event Panel Close? {
          n146 = event-data() -> ()  [unwired: 1 in, 1 out]
          n147 = event-data("Discard?"=TRUE) -> ()  [unwired: 1 in, 1 out]
        }
        event Key Down? {
          n148 = event-data() -> ()  [unwired: 1 in, 1 out]
          n149 = event-data() -> ()  [unwired: 2 in, 1 out]
        }
      }
    }
  }
  n150 = Release Queue(queue=w59) -> ()  [unwired: 2 in, 3 out]
